vi "Module - Report Generation.vi"(9 "Generate Report":bool, 10 "Stop":bool, 11 "Button":bool) -> (0 "Error Out":errorcluster)   [LabVIEW 2020]
uses:
  Control/State - Report Generation.ctl
  Control/Data Struc -Write Multiple Data.ctl
  Control/Data to Execute.ctl
  Control/Transaction Info.ctl
  Control/Product Info.ctl
  Control/Acceptance Criteria Info.ctl
  Control/Execution Info.ctl
  Control/Results Info.ctl
  Control/State - eFGV.ctl
  Control/State - FGV.ctl
  <vilib>/Utility/NIReport.llb/HTML Report Image Alignment.ctl
  Control/Data Struc - Image Report Setup.ctl
  Control/Operation - Report Generation.ctl
  <vilib>/Utility/file.llb/Read Delimited Spreadsheet (string).vi
  <vilib>/Utility/NIReport.llb/NI_ReportGenerationCore.lvlib
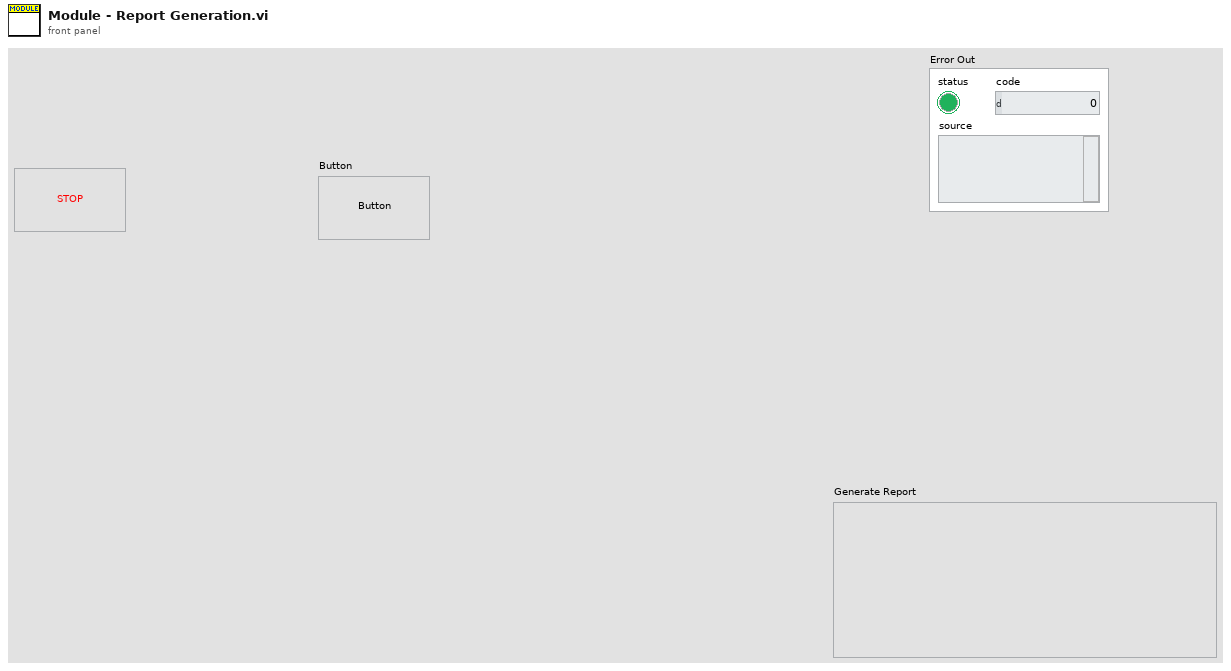
[diagram p1: front panel]
types:
  T1 = typedef "Data Struc -Write Multiple Data.ctl" = cluster{"column headers":string[], "text data":string[][], "worksheet index (0)":i32, "MS Office parameters":cluster{"position (excel)":cluster{"row":i32, "column":i32}, "name (excel)":string, "bookmark (word)":string}}
  T2 = typedef "Data to Execute.ctl" = cluster{"Transaction Info":T3, "Product Info":T4, "Misc - Additional Refs":string[][], "Misc - Sensors":string[][], "Misc - Tools":string[][], "Acceptance Criteria Info":T5, "Execution Info":T6, "Results Info":T7, "Notes":string}
  T3 = typedef "Transaction Info.ctl" = cluster{"Transaction Number":u32, "Order Number":u32, "Quantity":u16, "Customer":u32, "Customer Description":string, "Project":string, "Sales Order":u32, "Material":u32, "Material Description":string, "Rework":bool, "NCR No.":string, "Ref Order No.":dbl, "Item No.":u32, "BOM Rev.":dbl}
  T4 = typedef "Product Info.ctl" = cluster{"Product Category":string, "Procedure No./Ref.":string, "Test System":string, "Test System Description":string, "Working Pressure":string, "Pressure Unit":string, "Rev.":string, "PSL":string}
  T5 = typedef "Acceptance Criteria Info.ctl" = cluster{"Max Start Hold Pressure":dbl, "Enum.Max Start Hold Pressure":enum16{"%", "psi"}, "Permitted Hold Pressure Drop":dbl, "Enum.Permitted Hold Pressure Drop":enum16{"%", "psi"}}
  T6 = typedef "Execution Info.ctl" = cluster{"Auto Set Marker":bool, "Auto Stop Test":bool}
  T7 = typedef "Results Info.ctl" = cluster{"ListBox.Output Set":string, "Output Set Description":string}
  T8 = cluster{"T_Out":i32, "Report Folder Path":path, "Write Multiple Data":T1[], "Result Folder Path":path, "Report Template Path":path, "Data to Execute":T2, "Setup data":string[], "Execute Data":string[], "Event Ref":refnum<event-registration>, "Data To Report":cluster{"Execute Data":string[], "Sequence no":string}}
  T9 = typedef "State - Report Generation.ctl" = enum16{"Init", "Register Event", "Init File Directory", "Idle", "Transaction Info Data", "Product Data info", "Execute Info", "Execute Data", "Report Gen Setup", "Read Datalog", "Generate Report", "Save Image", "Close"}
  T10 = typedef "State - FGV.ctl" = enum16{"Write", "Read"}
  T11 = typedef "Operation - Report Generation.ctl" = enum16{"Get List Setup", "Save Image", "Generate Report"}
  T12 = typedef "Data Struc - Image Report Setup.ctl" = cluster{"alignment (default)":T13, "path or URL of image":path[], "worksheet index (0)":i32, "caption or alternative string":string[]}
  T13 = typedef "NI_ReportGenerationCore.lvlib/HTML Report Image Alignment.ctl" = enum16{"(default)", "LEFT", "RIGHT", "TOP", "TEXTTOP", "MIDDLE", "ABSMIDDLE", "BASELINE", "BOTTOM", "ABSBOTTOM"}
  T14 = typedef "State - eFGV.ctl" = enum16{"Init", "Read", "Write", "Exit"}
  T15 = enum32{"invalid app kind", "Development System", "Run Time System", "Student Edition", "Embedded LabVIEW", "Evaluation", "Custom"}
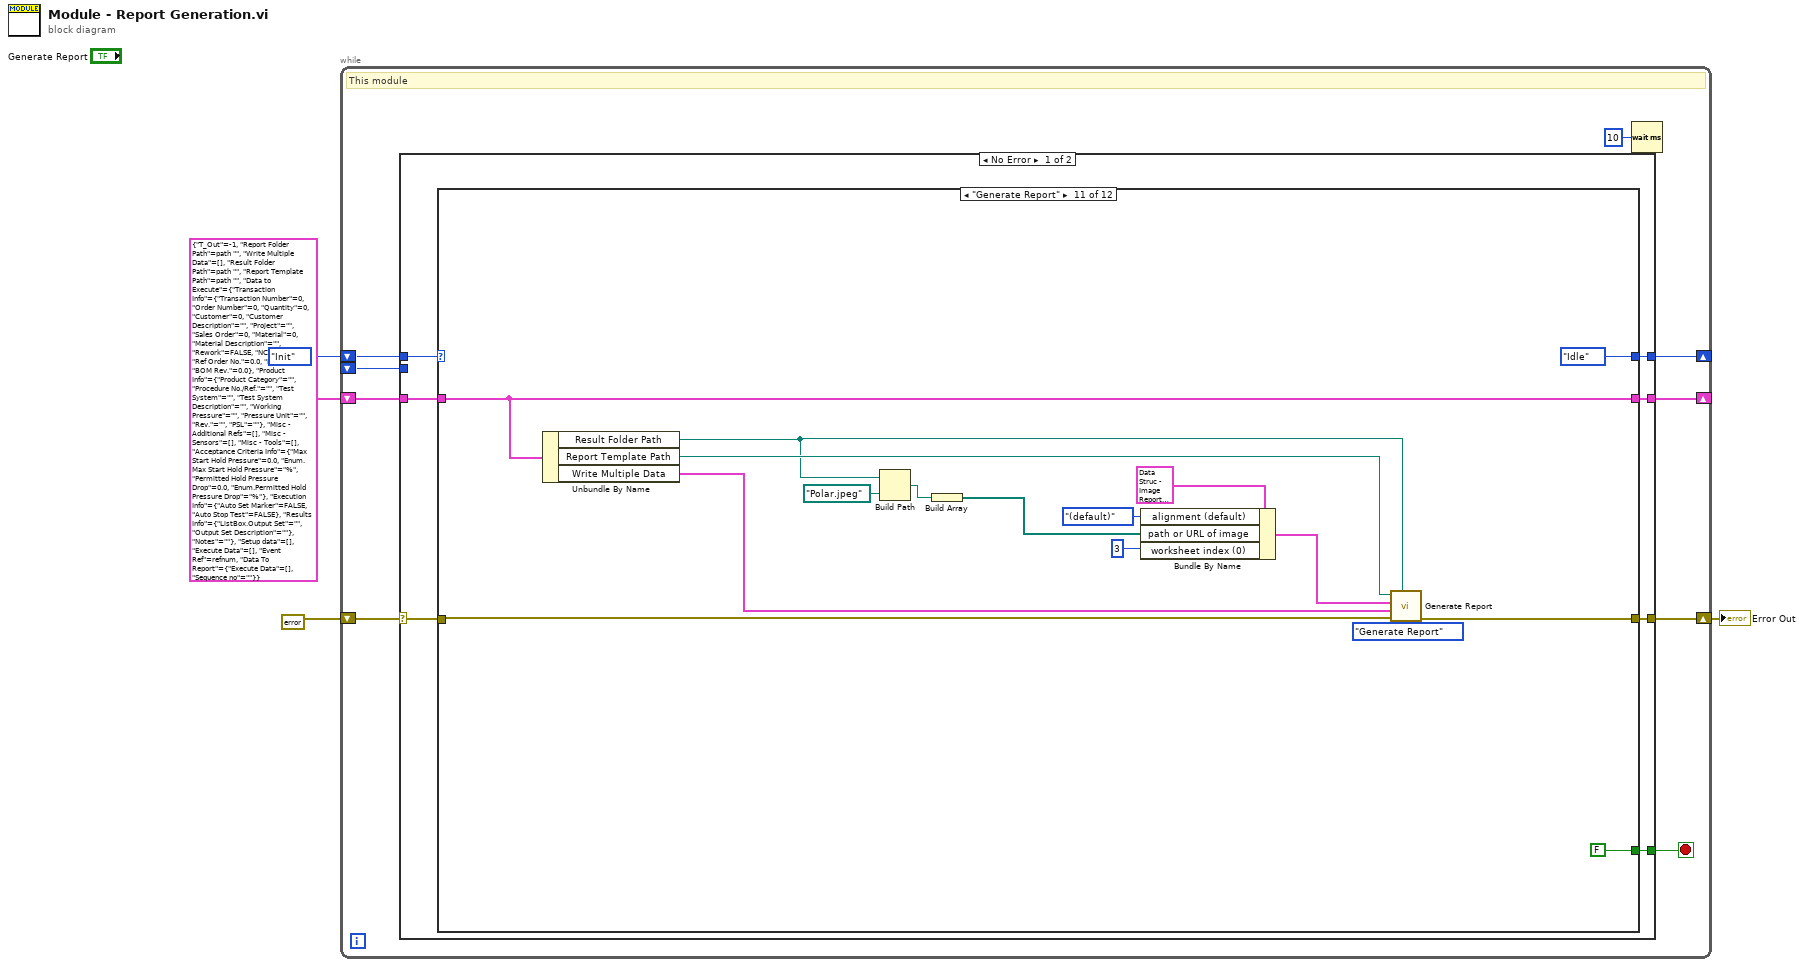
[diagram p0: block diagram]
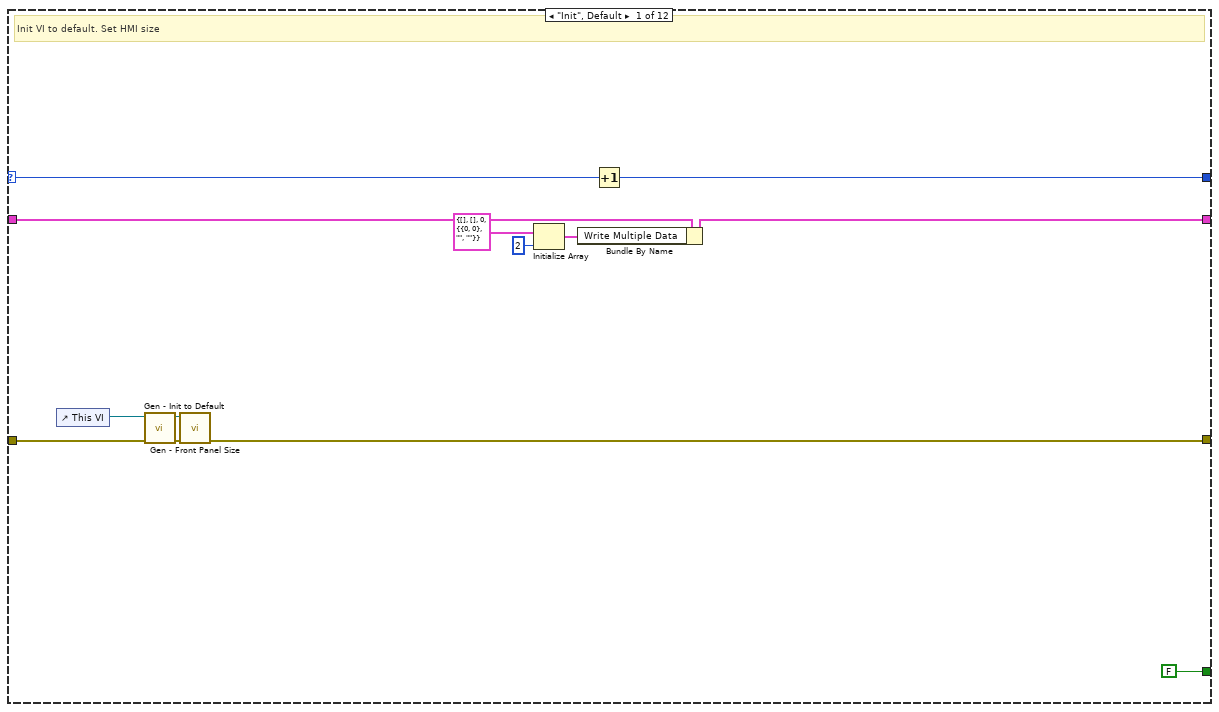
[diagram p2: hidden frame]
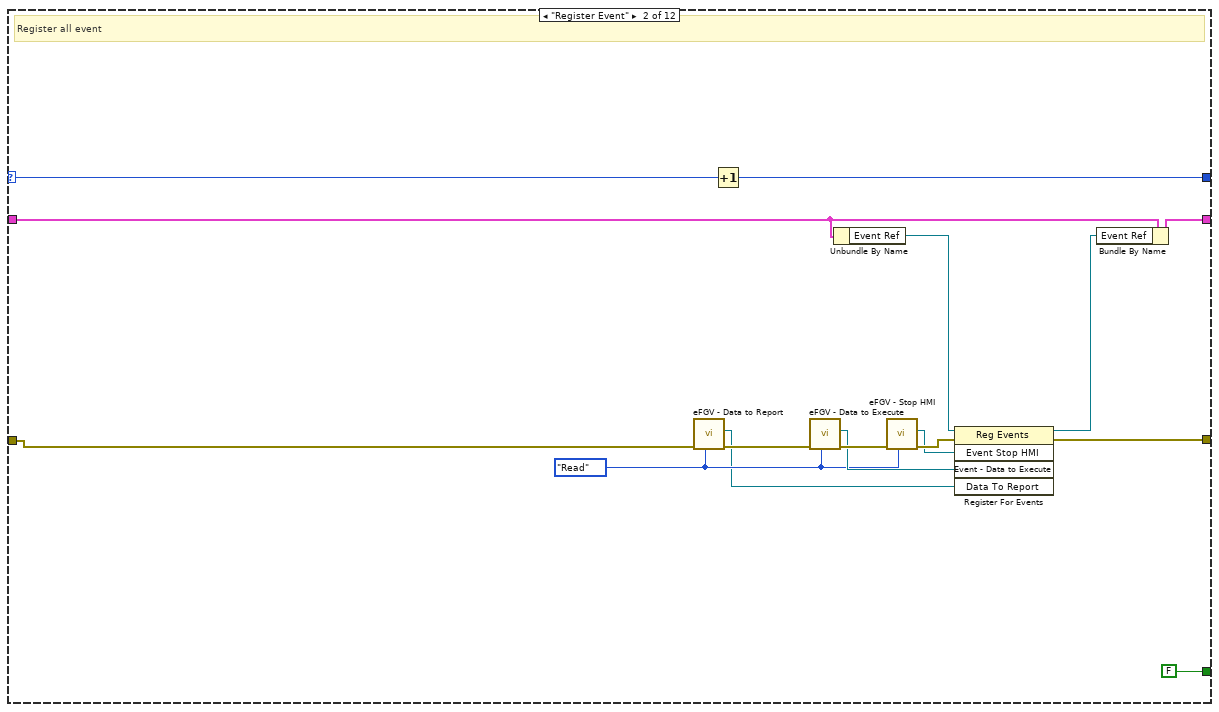
[diagram p3: hidden frame]
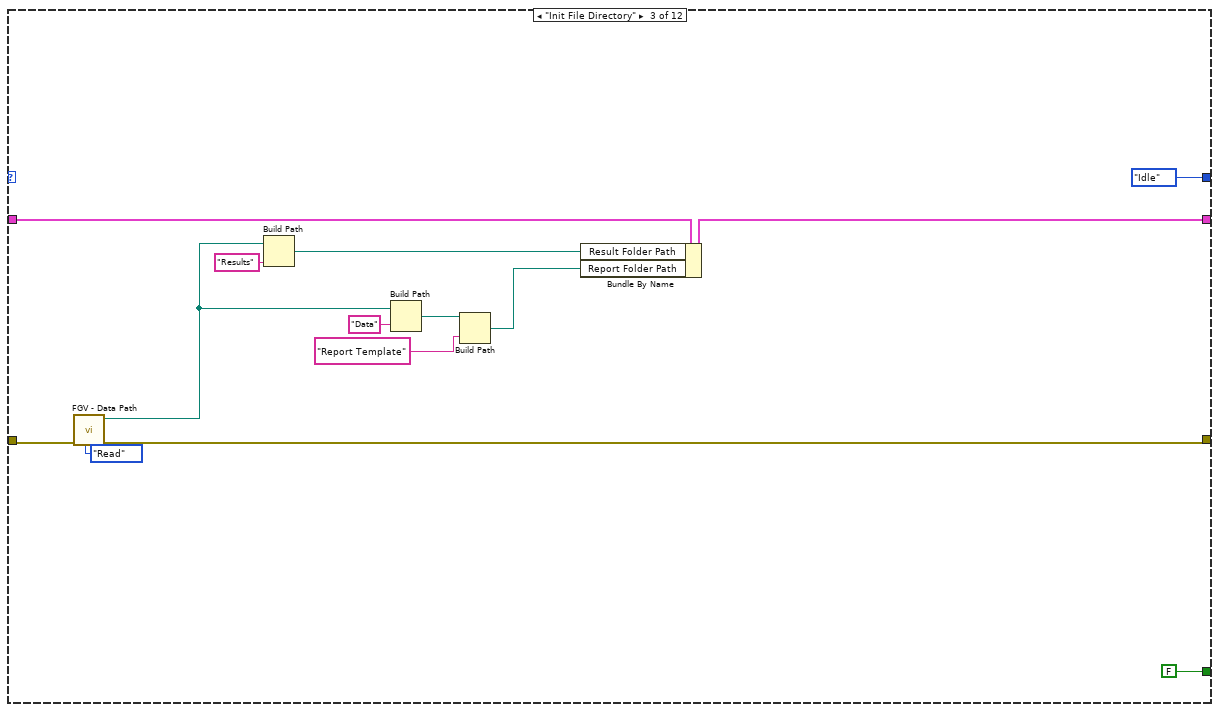
[diagram p4: hidden frame]
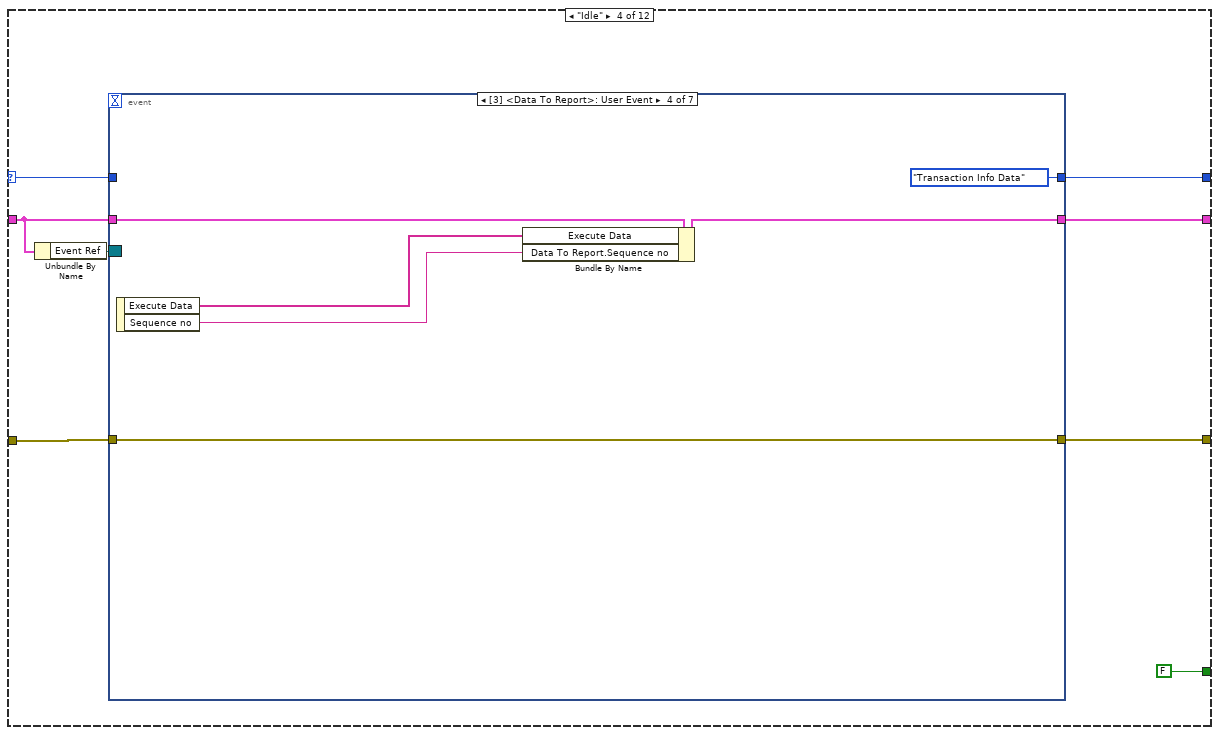
[diagram p5: hidden frame]
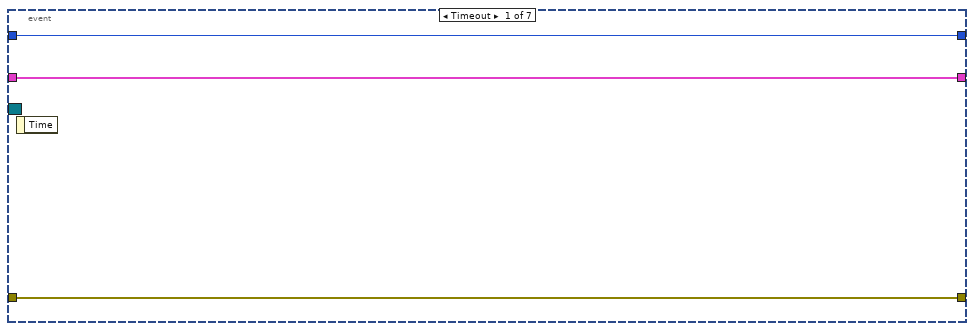
[diagram p6: hidden frame]
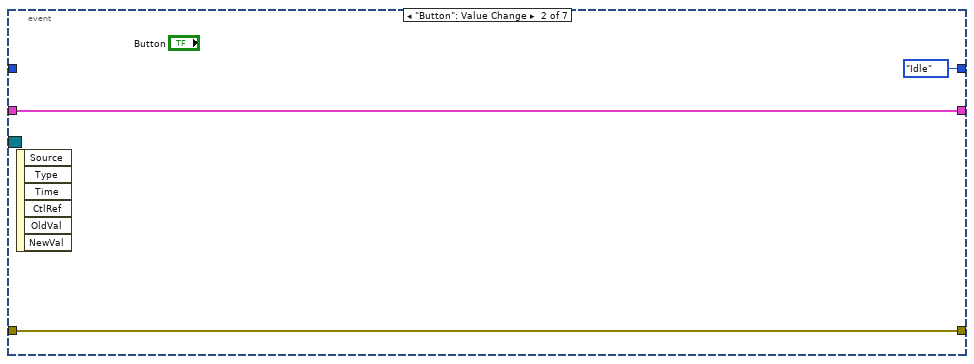
[diagram p7: hidden frame]
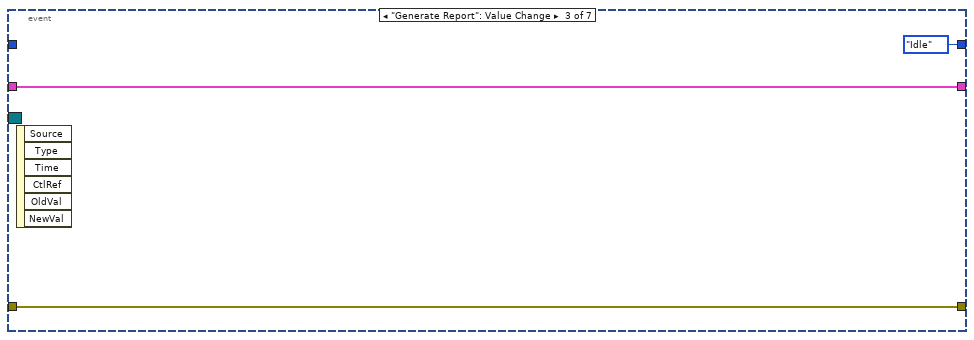
[diagram p8: hidden frame]
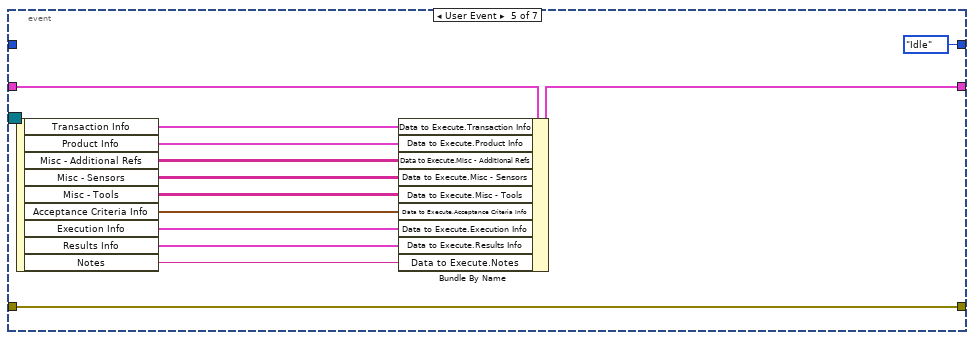
[diagram p9: hidden frame]
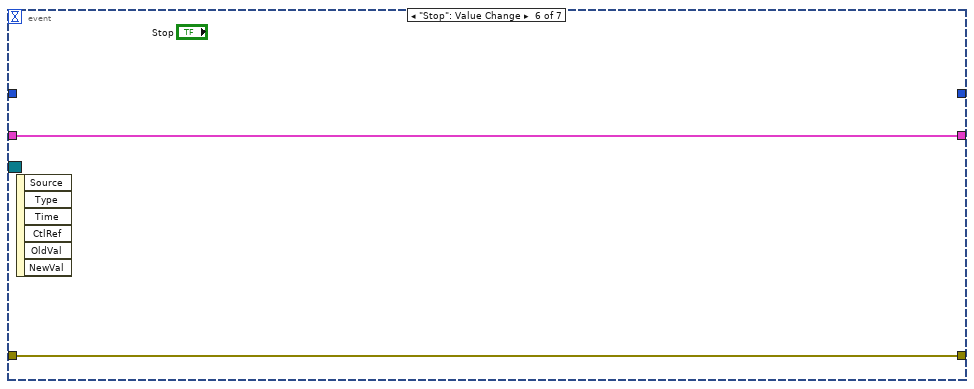
[diagram p10: hidden frame]
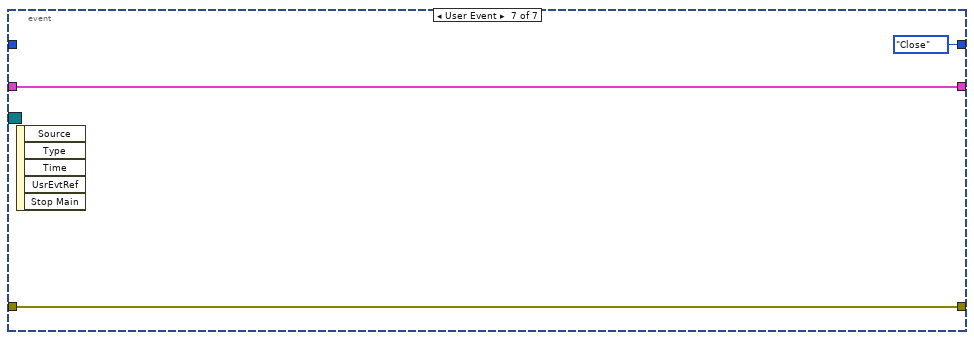
[diagram p11: hidden frame]
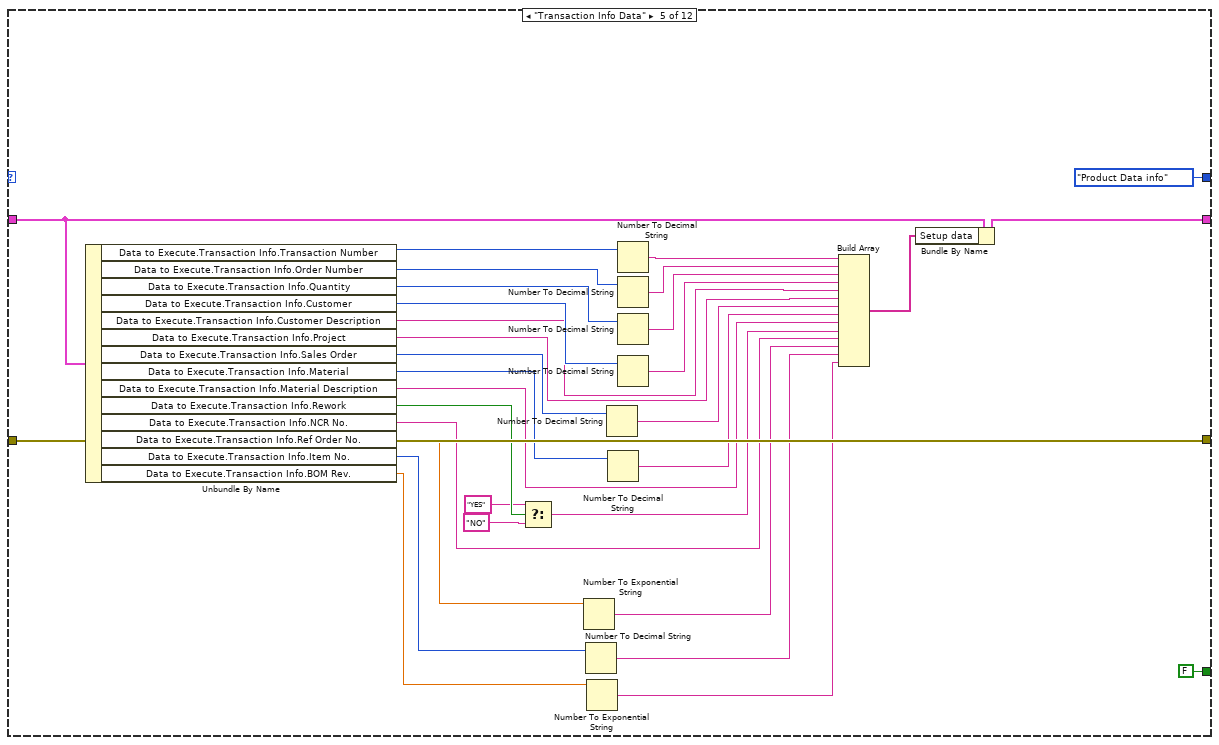
[diagram p12: hidden frame]
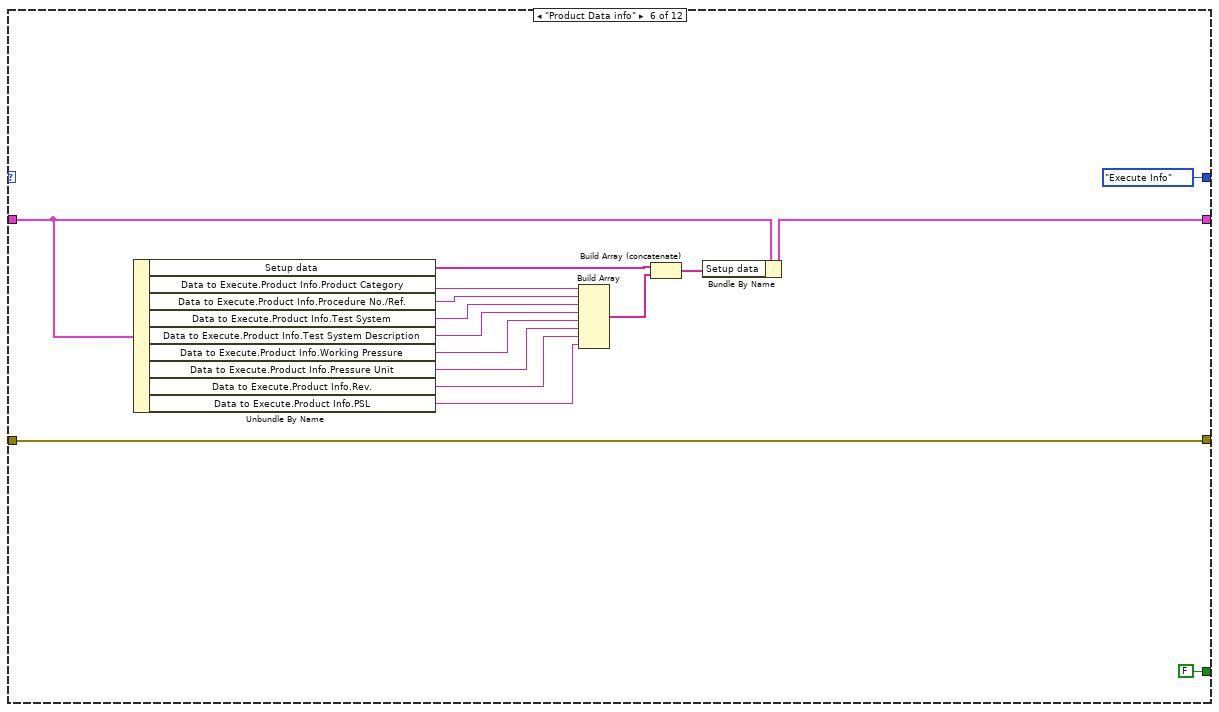
[diagram p13: hidden frame]
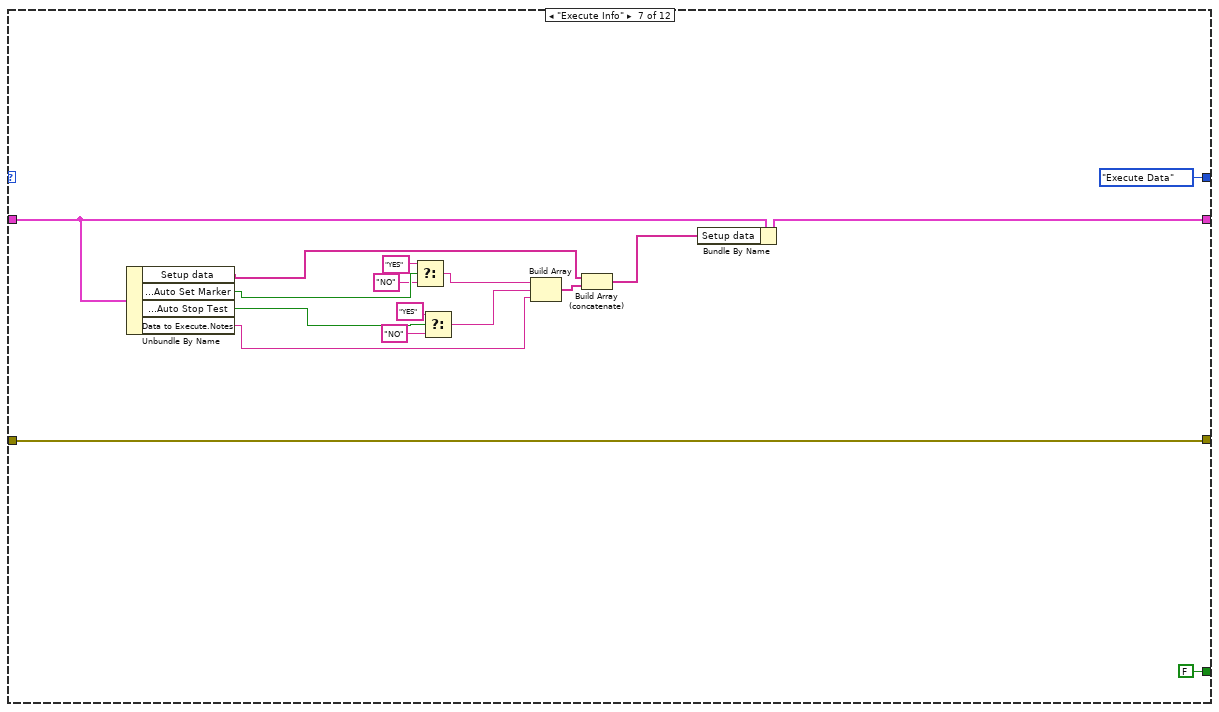
[diagram p14: hidden frame]
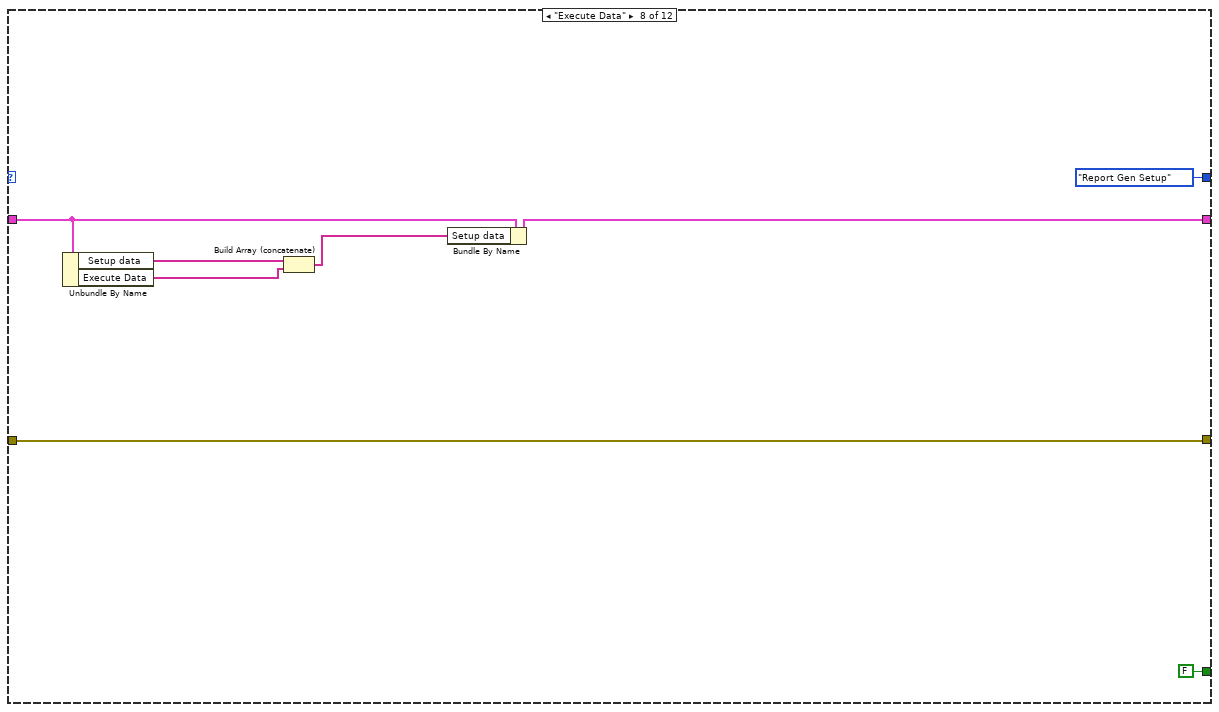
[diagram p15: hidden frame]
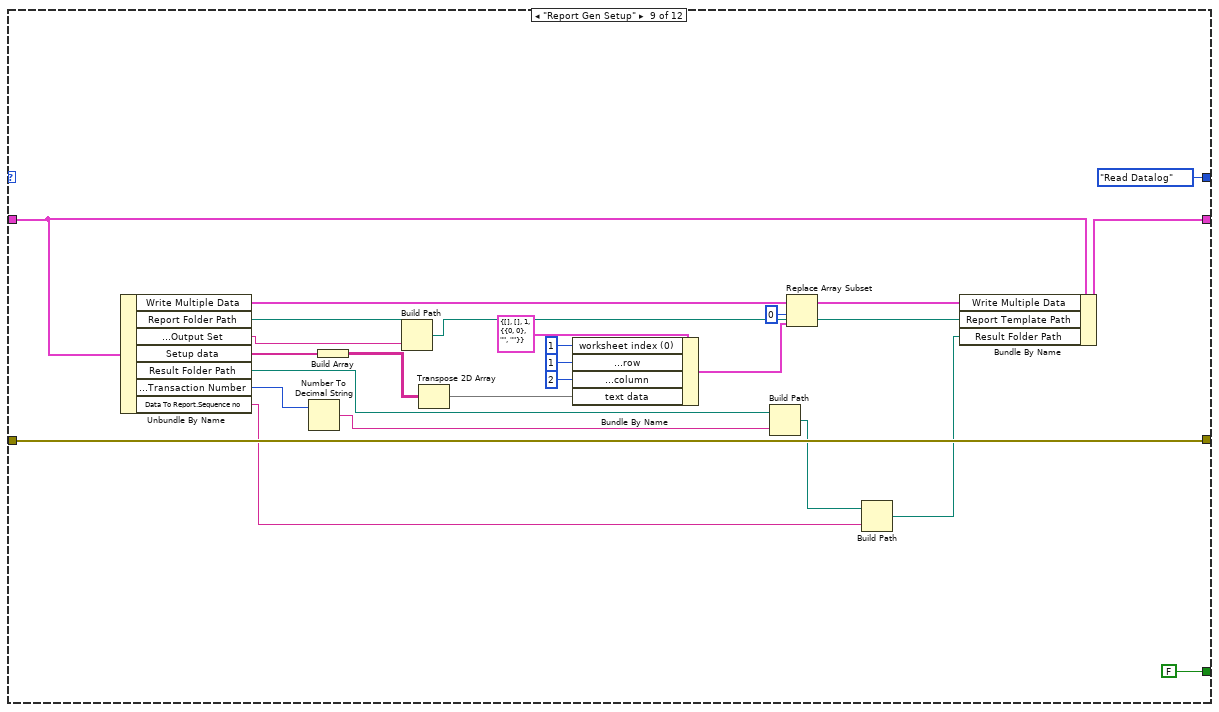
[diagram p16: hidden frame]
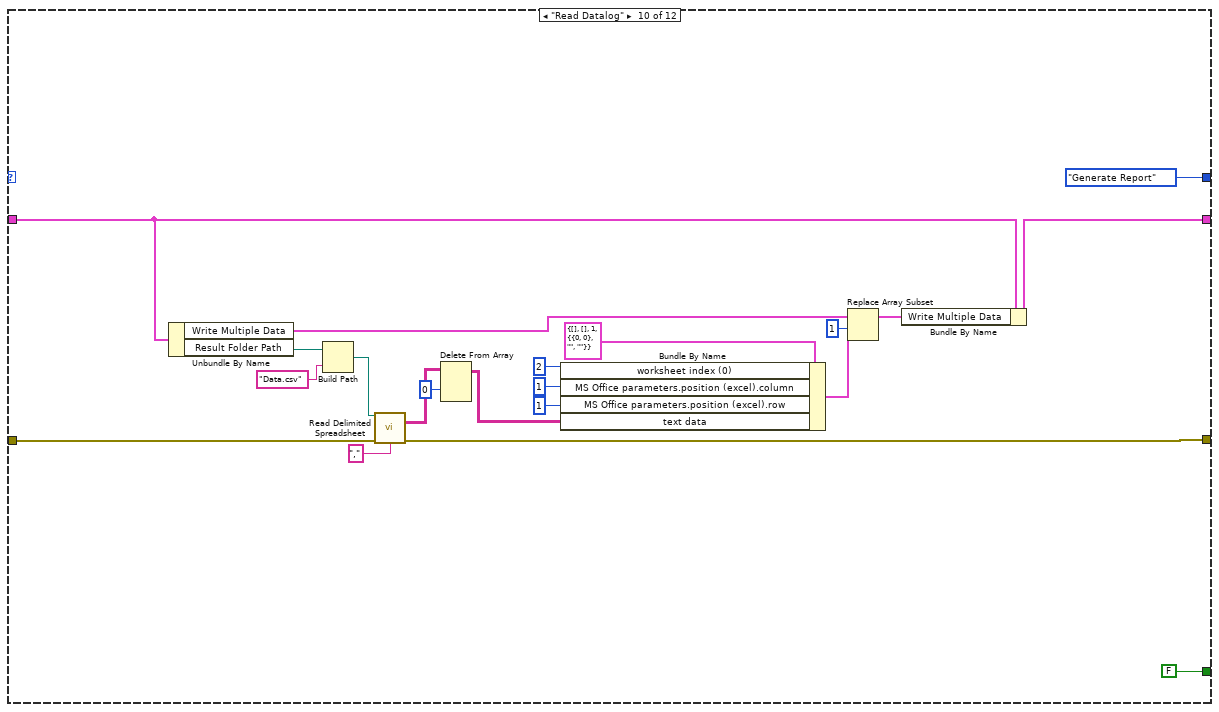
[diagram p17: hidden frame]
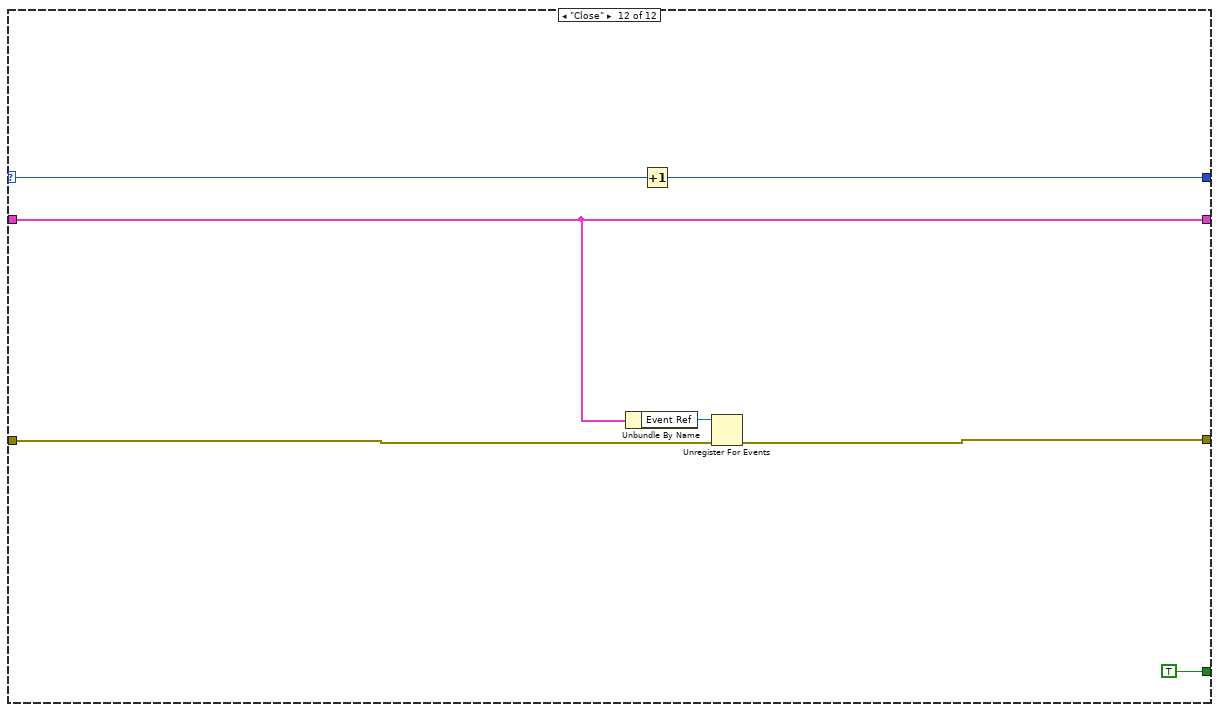
[diagram p18: hidden frame]
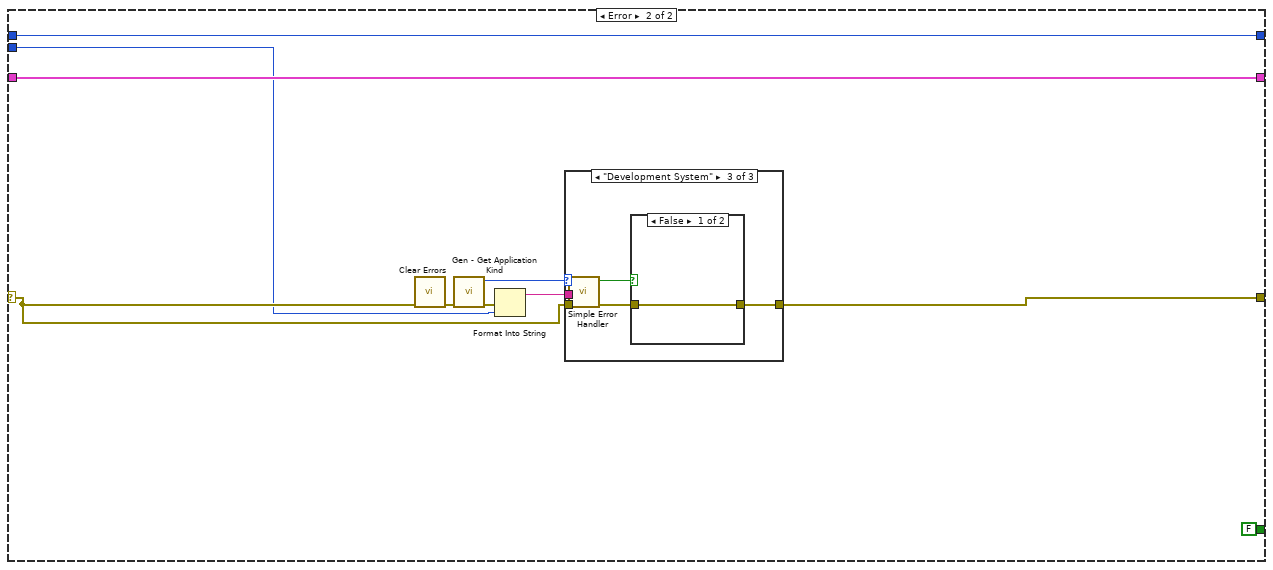
[diagram p19: hidden frame]
diagram:
  w1 = State_-_Report_Generation."Init"
  n1 = while {
    shift-right: [w9] -> _
    shift-left: w1 -> [w11]
    shift-right: [w12] -> w3
    shift-left: errorcluster {"status"=FALSE, "code"=0, "source"=""} ("Error In") -> [w13]
    shift-right: [w7] -> _
    shift-left: T8 {"T_Out"=-1, "Report Folder Path"=path "", "Write Multiple Data"=[], "Result Folder Path"=path "", "Report Template Path"=path "", "Data to Execute"={"Transaction Info"={"Transaction Number"=0, "Order Number"=0, "Quantity"=0, "Customer"=0, "Customer Description"="", "Project"="", "Sales Order"=0, "Material"=0, "Material Description"="", "Rework"=FALSE, "NCR No."="", "Ref Order No."=0.0, "Item No."=0, "BOM Rev."=0.0}, "Product Info"={"Product Category"="", "Procedure No./Ref."="", "Test System"="", "Test System Description"="", "Working Pressure"="", "Pressure Unit"="", "Rev."="", "PSL"=""}, "Misc - Additional Refs"=[], "Misc - Sensors"=[], "Misc - Tools"=[], "Acceptance Criteria Info"={"Max Start Hold Pressure"=0.0, "Enum.Max Start Hold Pressure"=enum."%", "Permitted Hold Pressure Drop"=0.0, "Enum.Permitted Hold Pressure Drop"=enum."%"}, "Execution Info"={"Auto Set Marker"=FALSE, "Auto Stop Test"=FALSE}, "Results Info"={"ListBox.Output Set"="", "Output Set Description"=""}, "Notes"=""}, "Setup data"=[], "Execute Data"=[], "Event Ref"=refnum, "Data To Report"={"Execute Data"=[], "Sequence no"=""}} -> [w8]
    shift-left: w1 -> [w5]
    stop <- w10 stop-if-true
    # "This module"
    n2 = case shown="No Error" w13 {
      selector: w13 -> [w19 w254]
      tunnel: w11 -> [w18 w251]
      tunnel: [w20 w255] -> w12
      tunnel: [w17 FALSE] -> w10
      tunnel: [w16 w251] -> w9
      tunnel: w8 -> [w15 w250]
      tunnel: [w14 w250] -> w7
      tunnel: w5 -> [_ w247]
      frame No Error {
        n3 = case shown="\"Generate Report\"" w18 {
          selector: w18 -> [w26 w42 _ w66 _ _ _ _ _ _ _ w244]
          tunnel: [w31 w49 w62 w71 w136 w152 w169 w177 w202 w222 w239 w245] -> w20
          tunnel: w19 -> [w33 w39 w63 w70 w136 w152 w169 w177 w202 w223 w238 w246]
          tunnel: [FALSE FALSE FALSE FALSE FALSE FALSE FALSE FALSE FALSE FALSE FALSE TRUE] -> w17
          tunnel: [w25 w41 State_-_Report_Generation."Idle" w68 State_-_Report_Generation."Product Data info" State_-_Report_Generation."Execute Info" State_-_Report_Generation."Execute Data" State_-_Report_Generation."Report Gen Setup" State_-_Report_Generation."Read Datalog" State_-_Report_Generation."Generate Report" State_-_Report_Generation."Idle" w240] -> w16
          tunnel: w15 -> [w30 w44 w61 w65 w133 w150 w167 w175 w200 w219 w235 w242]
          tunnel: [w24 w43 w56 w67 w106 w139 w155 w172 w199 w214 w235 w242] -> w14
          frame "Init", Default {
            # "Init VI to default. Set HMI size"
            n4 = control-ref of="This VI"() -> (w28:refnum<vi>)
            n5 = call "Gen - Init to Default.vi"("Error in"=w33, "This VI"=w28) -> ("Error out"=w32:errorcluster, "This VI Copy"=w27:refnum<vi>)  [unwired: 8 in]
            n6 = call "Gen - Front Panel Size.vi"("Error In"=w32, "This VI"=w27) -> ("Error Out"=w31:errorcluster)  [unwired: 9 in]
            n7 = Initialize Array(T1 {"column headers"=[], "text data"=[], "worksheet index (0)"=0, "MS Office parameters"={"position (excel)"={"row"=0, "column"=0}, "name (excel)"="", "bookmark (word)"=""}} ("Write Multiple Data"), 2 ("dimension size")) -> (w21:T1[])
            n8 = Bundle By Name(cluster=w30, "Write Multiple Data"=w21) -> (w24:T8)
            n9 = Increment(x=w26) -> (x+1=w25:T9)
          }
          frame "Register Event" {
            w37 = State_-_eFGV."Read" ("Action")
            # "Register all event"
            n10 = call "eFGV - Data to Report.vi"("Action"=w37, "Error In"=w39) -> ("Error Out"=w38:errorcluster, "Data To Report"=w36:refnum<user-event>)  [unwired: 8 in]
            n11 = Increment(x=w42) -> (x+1=w41:T9)
            n12 = call "eFGV - Data to Execute.vi"("Action"=w37, "Error In"=w38) -> ("Error Out"=w47:errorcluster, "Event - Data to Execute"=w40:refnum<user-event>)  [unwired: 8 in]
            n13 = Unbundle By Name(w44) -> ("Event Ref"=w35:refnum<event-registration>)
            n14 = call "eFGV - Stop HMI.vi"("Action"=w37, "Error In"=w47) -> ("Error Out"=w48:errorcluster, "Event Stop HMI"=w45:refnum<user-event>)  [unwired: 7 in, 1 out]
            n15 = register-events(reference=w35, error in=w48, w45, w40, w36) -> (reference out=w34:refnum<event-registration>, error out=w49:errorcluster)
            n16 = Bundle By Name(cluster=w44, "Event Ref"=w34) -> (w43:T8)
          }
          frame "Init File Directory" {
            n17 = call "FGV - Data Path.vi"("FGV State"=State_-_FGV."Read", "Error In"=w63) -> ("Error Out"=w62:errorcluster, "Path Out"=w51:path)  [unwired: 8 in]
            n18 = Build Path(base path=w51, name or relative path="Results") -> (appended path=w55:path)
            n19 = Build Path(base path=w51, name or relative path="Data") -> (appended path=w53:path)
            n20 = Build Path(base path=w53, name or relative path="Report Template") -> (appended path=w50:path)
            n21 = Bundle By Name(cluster=w61, "Result Folder Path"=w55, "Report Folder Path"=w50) -> (w56:T8)
          }
          frame "Idle" {
            n22 = Unbundle By Name(w65) -> ("Event Ref"=w64:refnum<event-registration>)
            n23 = event shown="[3] <Data To Report>: User Event" {
              selector: w64 -> [_ _ _ _ _ _ _]
              dyn-events: _ -> [_ _ _ _ _ _ _]
              timeout: _ -> [_ _ _ _ _ _ _]
              tunnel: [w74 w77 w80 w86 w99 w101 w104] -> w71
              tunnel: w70 -> [w74 w77 w80 w86 w99 w101 w104]
              tunnel: [w72 State_-_Report_Generation."Idle" State_-_Report_Generation."Idle" State_-_Report_Generation."Transaction Info Data" State_-_Report_Generation."Idle" _ State_-_Report_Generation."Close"] -> w68
              tunnel: [w73 w76 w79 w83 w96 w100 w103] -> w67
              tunnel: w65 -> [w73 w76 w79 w85 w98 w100 w103]
              tunnel: w66 -> [w72 _ _ _ _ _ _]
              event Timeout {
                n24 = event-data() -> ()  [unwired: 1 in, 1 out]
              }
              event "Button": Value Change {
                n25 = event-data() -> ()  [unwired: 1 in, 6 out]
              }
              event "Generate Report": Value Change {
                n26 = event-data() -> ()  [unwired: 1 in, 6 out]
              }
              event User Event {
                n27 = event-data() -> ("Execute Data"=w82:string[], "Sequence no"=w81:string)  [unwired: 1 in]
                n28 = Bundle By Name(cluster=w85, "Execute Data"=w82, "Data To Report.Sequence no"=w81) -> (w83:T8)
              }
              event User Event {
                n29 = event-data() -> ("Transaction Info"=w95:T3, "Product Info"=w87:T4, "Misc - Additional Refs"=w88:string[][], "Misc - Sensors"=w89:string[][], "Misc - Tools"=w90:string[][], "Acceptance Criteria Info"=w91:T5, "Execution Info"=w92:T6, "Results Info"=w93:T7, "Notes"=w94:string)  [unwired: 1 in]
                n30 = Bundle By Name(cluster=w98, "Data to Execute.Transaction Info"=w95, "Data to Execute.Product Info"=w87, "Data to Execute.Misc - Additional Refs"=w88, "Data to Execute.Misc - Sensors"=w89, "Data to Execute.Misc - Tools"=w90, "Data to Execute.Acceptance Criteria Info"=w91, "Data to Execute.Execution Info"=w92, "Data to Execute.Results Info"=w93, "Data to Execute.Notes"=w94) -> (w96:T8)
              }
              event "Stop": Value Change {
                n31 = event-data() -> ()  [unwired: 1 in, 6 out]
              }
              event User Event {
                n32 = event-data() -> ()  [unwired: 1 in, 5 out]
              }
            }
          }
          frame "Transaction Info Data" {
            n33 = Unbundle By Name(w133) -> ("Data to Execute.Transaction Info.Transaction Number"=w132:u32, "Data to Execute.Transaction Info.Order Number"=w131:u32, "Data to Execute.Transaction Info.Quantity"=w130:u16, "Data to Execute.Transaction Info.Customer"=w129:u32, "Data to Execute.Transaction Info.Customer Description"=w122:string, "Data to Execute.Transaction Info.Project"=w121:string, "Data to Execute.Transaction Info.Sales Order"=w128:u32, "Data to Execute.Transaction Info.Material"=w127:u32, "Data to Execute.Transaction Info.Material Description"=w118:string, "Data to Execute.Transaction Info.Rework"=w117:bool, "Data to Execute.Transaction Info.NCR No."=w113:string, "Data to Execute.Transaction Info.Ref Order No."=w112:dbl, "Data to Execute.Transaction Info.Item No."=w110:u32, "Data to Execute.Transaction Info.BOM Rev."=w107:dbl)
            n34 = Select(t="YES", s=w117, f="NO") -> (s? t:f=w114:string)
            n35 = Number To Exponential String(number=w112) -> (E-format string=w111:string)  [unwired: 3 in]
            n36 = Number To Decimal String(number=w110) -> (decimal integer string=w109:string)  [unwired: 1 in]
            n37 = Number To Exponential String(number=w107) -> (E-format string=w108:string)  [unwired: 3 in]
            n38 = Number To Decimal String(number=w128) -> (decimal integer string=w120:string)  [unwired: 1 in]
            n39 = Number To Decimal String(number=w127) -> (decimal integer string=w119:string)  [unwired: 1 in]
            n40 = Number To Decimal String(number=w132) -> (decimal integer string=w126:string)  [unwired: 1 in]
            n41 = Number To Decimal String(number=w131) -> (decimal integer string=w125:string)  [unwired: 1 in]
            n42 = Number To Decimal String(number=w130) -> (decimal integer string=w124:string)  [unwired: 1 in]
            n43 = Number To Decimal String(number=w129) -> (decimal integer string=w123:string)  [unwired: 1 in]
            n44 = Build Array(w126, w125, w124, w123, w122, w121, w120, w119, w118, w114, w113, w111, w109, w108) -> (w105:string[])
            n45 = Bundle By Name(cluster=w133, "Setup data"=w105) -> (w106:T8)
          }
          frame "Product Data info" {
            n46 = Unbundle By Name(w150) -> ("Setup data"=w141:string[], "Data to Execute.Product Info.Product Category"=w149:string, "Data to Execute.Product Info.Procedure No./Ref."=w148:string, "Data to Execute.Product Info.Test System"=w147:string, "Data to Execute.Product Info.Test System Description"=w146:string, "Data to Execute.Product Info.Working Pressure"=w145:string, "Data to Execute.Product Info.Pressure Unit"=w144:string, "Data to Execute.Product Info.Rev."=w143:string, "Data to Execute.Product Info.PSL"=w142:string)
            n47 = Build Array(w149, w148, w147, w146, w145, w144, w143, w142) -> (w140:string[])
            n48 = Build Array (concatenate)(w141, w140) -> (w138:string[])
            n49 = Bundle By Name(cluster=w150, "Setup data"=w138) -> (w139:T8)
          }
          frame "Execute Info" {
            n50 = Unbundle By Name(w167) -> ("Setup data"=w156:string[], "Data to Execute.Execution Info.Auto Set Marker"=w166:bool, "Data to Execute.Execution Info.Auto Stop Test"=w165:bool, "Data to Execute.Notes"=w158:string)
            n51 = Select(t="YES", s=w166, f="NO") -> (s? t:f=w160:string)
            n52 = Select(t="YES", s=w165, f="NO") -> (s? t:f=w159:string)
            n53 = Build Array(w160, w159, w158) -> (w157:string[])
            n54 = Build Array (concatenate)(w156, w157) -> (w154:string[])
            n55 = Bundle By Name(cluster=w167, "Setup data"=w154) -> (w155:T8)
          }
          frame "Execute Data" {
            n56 = Unbundle By Name(w175) -> ("Setup data"=w174:string[], "Execute Data"=w173:string[])
            n57 = Build Array (concatenate)(w174, w173) -> (w171:string[])
            n58 = Bundle By Name(cluster=w175, "Setup data"=w171) -> (w172:T8)
          }
          frame "Report Gen Setup" {
            n59 = Unbundle By Name(w200) -> ("Write Multiple Data"=w198:T1[], "Report Folder Path"=w190:path, "Data to Execute.Results Info.ListBox.Output Set"=w185:string, "Setup data"=w188:string[], "Result Folder Path"=w182:path, "Data to Execute.Transaction Info.Transaction Number"=w184:u32, "Data To Report.Sequence no"=w179:string)
            n60 = Number To Decimal String(number=w184) -> (decimal integer string=w183:string)  [unwired: 1 in]
            n61 = Build Array(w188) -> (w187:string[][])
            n62 = Build Path(base path=w190, name or relative path=w185) -> (appended path=w186:path)
            n63 = Transpose 2D Array(2D array=w187) -> (transposed array=w178:string[][])
            n64 = Bundle By Name(cluster=T1 {"column headers"=[], "text data"=[], "worksheet index (0)"=1, "MS Office parameters"={"position (excel)"={"row"=0, "column"=0}, "name (excel)"="", "bookmark (word)"=""}} ("new element/subarray"), "worksheet index (0)"=1, "MS Office parameters.position (excel).row"=1, "MS Office parameters.position (excel).column"=2, "text data"=w178) -> (w194:T1)
            n65 = Build Path(base path=w182, name or relative path=w183) -> (appended path=w181:path)
            n66 = Replace Array Subset(array=w198, new element=w194, index=0) -> (w197:T1[])
            n67 = Build Path(base path=w181, name or relative path=w179) -> (appended path=w180:path)
            n68 = Bundle By Name(cluster=w200, "Write Multiple Data"=w197, "Report Template Path"=w186, "Result Folder Path"=w180) -> (w199:T8)
          }
          frame "Read Datalog" {
            n69 = Unbundle By Name(w219) -> ("Write Multiple Data"=w218:T1[], "Result Folder Path"=w208:path)
            n70 = Build Path(base path=w208, name or relative path="Data.csv") -> (appended path=w205:path)
            n71 = call-poly <vilib>:"Read Delimited Spreadsheet.vi"("file path (dialog if empty)"=w205, "error in (no error)"=w223, "delimiter (\\t)"="," ("delimiter (\\t)")) -> ("all rows"=w206:string[][], "error out"=w222:errorcluster)  [unwired: 7 in, 4 out]
            n72 = Delete From Array(array=w206, index (row)=0) -> (array with subset deleted=w203:string[][])  [unwired: 2 in, 1 out]
            n73 = Bundle By Name(cluster=T1 {"column headers"=[], "text data"=[], "worksheet index (0)"=1, "MS Office parameters"={"position (excel)"={"row"=0, "column"=0}, "name (excel)"="", "bookmark (word)"=""}} ("new element/subarray"), "worksheet index (0)"=2, "MS Office parameters.position (excel).column"=1, "MS Office parameters.position (excel).row"=1, "text data"=w203) -> (w216:T1)
            n74 = Replace Array Subset(array=w218, new element=w216, index=1) -> (w213:T1[])
            n75 = Bundle By Name(cluster=w219, "Write Multiple Data"=w213) -> (w214:T8)
          }
          frame "Generate Report" {
            n76 = Unbundle By Name(w235) -> ("Result Folder Path"=w227:path, "Report Template Path"=w234:path, "Write Multiple Data"=w228:T1[])
            n77 = Build Path(base path=w227, name or relative path=path "Polar.jpeg") -> (appended path=w225:path)
            n78 = Build Array(w225) -> (w224:path[])
            n79 = Bundle By Name(cluster=T12 {"alignment (default)"=enum."(default)", "path or URL of image"=[path "C:/Users/hasni/Documents/g159-one-subsea-test-pressure-monitoring-system/VI/HMI/Data/Data/Polar Plot/04012022_154036.jpeg"], "worksheet index (0)"=3, "caption or alternative string"=[]} ("Image Report Setup"), "alignment (default)"=HTML_Report_Image_Alignment."(default)", "path or URL of image"=w224, "worksheet index (0)"=3) -> (w230:T12)
            n80 = call "Generate Report.vi"(6:Operation_-_Report_Generation."Generate Report", "report file path"=w227, "error in (no error)"=w238, "Write Multiple Data"=w228, "Image Report Setup"=w230, "template (empty)"=w234) -> ("error out"=w239:errorcluster)  [unwired: 4 in, 1 out]
          }
          frame "Close" {
            n81 = Unbundle By Name(w242) -> ("Event Ref"=w241:refnum<event-registration>)
            n82 = Increment(x=w244) -> (x+1=w240:T9)
            n83 = Unregister For Events(event registration refnum=w241, error in=w246) -> (error out=w245:errorcluster)
          }
        }
      }
      frame Error {
        n84 = call <vilib>:"Clear Errors.vi"("error in (no error)"=w254) -> ("error out"=w256:errorcluster)  [unwired: 5 in, 1 out]
        n85 = call "Gen - Get Application Kind.vi"("Error In"=w256) -> ("Error Out"=w253:errorcluster, "Application:Kind"=w249:T15)  [unwired: 9 in]
        n86 = Format Into String(error in=w253, w247) -> (resulting string=w248:string)  [unwired: 2 in, 1 out]
        n87 = case shown="\"Development System\"" w249 {
          tunnel: [w257 w262 w266] -> w255
          tunnel: w254 -> [w257 w261 w264]
          tunnel: w248 -> [_ w258 _]
          frame "invalid app kind", Default {
          }
          frame "Run Time System" {
            n88 = control-ref of="This VI"() -> (w259:refnum<vi>)
            n89 = call "eFGV - Generated Error.vi"("eFGV States"=State_-_eFGV."Write", "Error In"=w261, "State"=w258, "This VI"=w259) -> ("Error Out"=w262:errorcluster)  [unwired: 6 in, 1 out]
          }
          frame "Development System" {
            n90 = call <vilib>:"Simple Error Handler.vi"("error in (no error)"=w264) -> ("error?"=w263:bool, "error out"=w265:errorcluster)  [unwired: 4 in, 3 out]
            n91 = case shown="False" w263 {
              tunnel: [w267 w269] -> w266
              tunnel: w265 -> [w267 w268]
              frame False {
              }
              frame True {
                n92 = call <vilib>:"Clear Errors.vi"("error in (no error)"=w268) -> ("error out"=w269:errorcluster)  [unwired: 5 in, 1 out]
              }
            }
          }
        }
      }
    }
    n93 = Wait (ms)(milliseconds to wait=u32 10) -> ()  [unwired: 1 out]
  }
  "Error Out" <- w3
